vi "Stop process.vi"(8 "error in (no error)":errorcluster, 11 "GIS Printer in":refnum<class "GIS Printer.lvclass">) -> (0 "error out":errorcluster, 3 "GIS Printer out":refnum<class "GIS Printer.lvclass">)   [LabVIEW 2022 SP3, in "GIS Printer.lvclass"]
uses:
  GIS Printer.lvclass
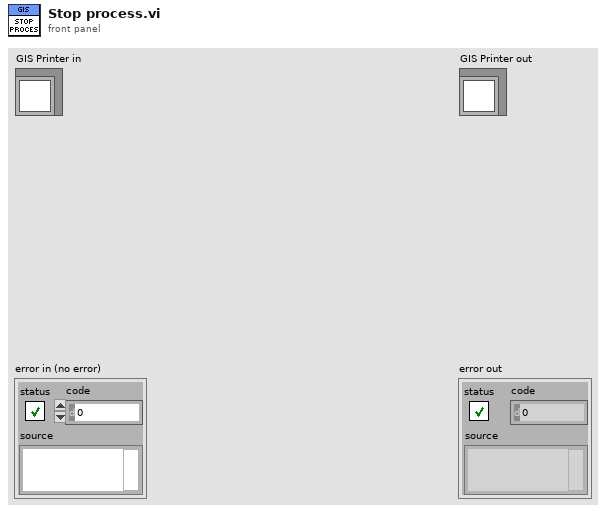
[diagram p1: front panel]
types:
  T1 = typedef "GIS Printer.lvclass/UserEvents.ctl" = cluster{"API Incoming Event":refnum<user-event>, "API Executed Event":refnum<user-event>, "API Return Event":refnum<user-event>, "Status Changed Event":refnum<user-event>, "Abort":refnum<user-event>, "stop process":refnum<user-event>, "GISPollStatus":refnum<user-event>, "GISHeadStatus":refnum<user-event>}
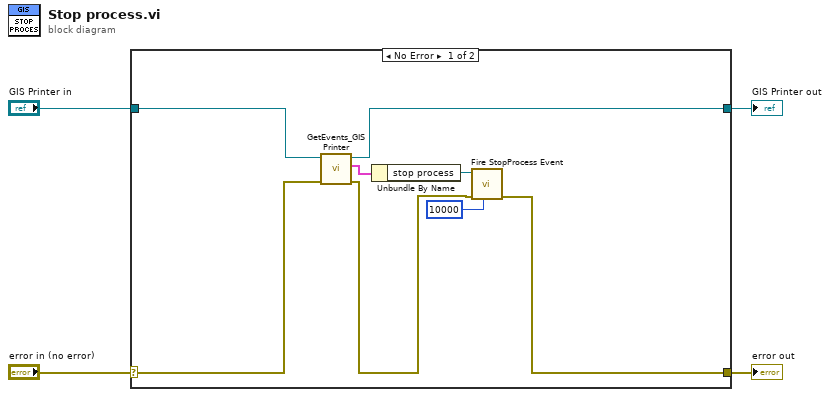
[diagram p0: block diagram]
diagram:
  n1 = case shown="No Error" "error in (no error)" {
    selector: "error in (no error)" -> [w6 w14]
    tunnel: [w9 w14] -> w3
    tunnel: [w8 w13] -> w1
    tunnel: "GIS Printer in" -> [w7 w13]
    frame No Error {
      n2 = call-dynamic "GetEvents_GIS Printer.vi"("error in (no error)"=w6, "TopLevel in"=w7) -> ("error out"=w5:errorcluster, "UserEvents"=w10:T1, "TopLevel out"=w8:refnum<class "GIS Printer.lvclass">)  [unwired: 7 in]
      n3 = Unbundle By Name(w10) -> ("stop process"=w11:refnum<user-event>)
      n4 = call "Fire StopProcess Event.vi"("timeout in ms (5000)"=10000, "error in (no error)"=w5, "Event in"=w11) -> ("error out"=w9:errorcluster)  [unwired: 5 in, 3 out]
    }
    frame Error {
    }
  }
  "error out" <- w3
  "GIS Printer out" <- w1
